vi "serpConfig.vi"() -> ()   [LabVIEW 2020]
panel:
  in  "VISA Aliases":string[](array[string])
  in  "delay break ?":bool=TRUE
  in  "specific reset ?":bool=TRUE
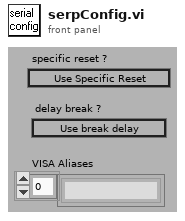
[diagram p1: front panel]
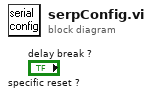
[diagram p0: block diagram]
diagram:
